vi "Configure Secured TCP Client Certificate and Key.vi"(4 "password":string, 6 "format (PKCS#8 (PEM))":enum32{"PKCS#8 (PEM)", "PKCS#8 (DER)"}(ring), 8 "error in (no error)":errorcluster, 9 "Client Key":path, 10 "X.509 Certificate":path, 11 "Connection.TCP-TLS in":refnum<class "Connection.TCP-TLS.lvclass">) -> (0 "error out":errorcluster, 2 "Ready for SSL":bool, 3 "Connection.TCP-TLS out":refnum<class "Connection.TCP-TLS.lvclass">)   [LabVIEW 2020, in "Connection.TCP-TLS.lvclass"]
uses:
  Connection.TCP-TLS.lvclass
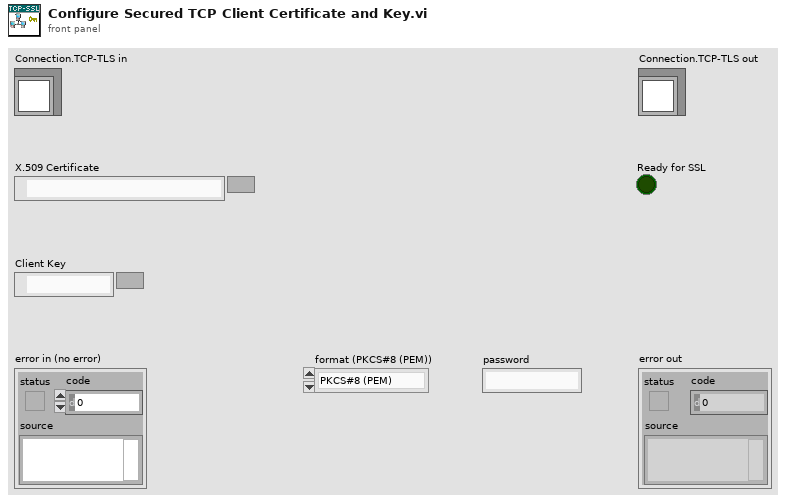
[diagram p1: front panel]
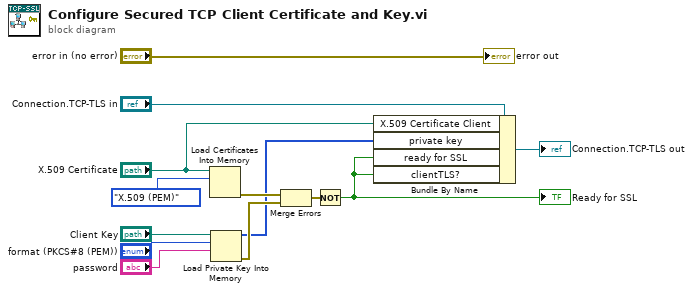
[diagram p0: block diagram]
diagram:
  n1 = Load Certificates Into Memory(10:enum32{"X.509 (PEM)"}."X.509 (PEM)" ("format"), 11:"X.509 Certificate") -> (0:w8:errorcluster)  [unwired: 1 in, 1 out]
  n2 = Load Private Key Into Memory(9:"password", 10:"format (PKCS#8 (PEM))", 11:"Client Key") -> (0:w7:errorcluster, 3:w4:u8[])  [unwired: 1 in]
  n3 = Merge Errors(w8, w7) -> (w9:errorcluster)
  n4 = Not(x=w9) -> (.not. x?=w1:bool)
  "Ready for SSL" <- w1
  n5 = Bundle By Name(cluster="Connection.TCP-TLS in", "X.509 Certificate Client"="X.509 Certificate", "private key"=w4, "ready for SSL"=w1, "clientTLS?"=w1) -> (→"Connection.TCP-TLS out":refnum<class "Connection.TCP-TLS.lvclass">)
  "error out" <- "error in (no error)"
